vi "Sampling to Loop ms.vi"(4 "Sampling Config":T1) -> (7 "Loop Timeout ms":i32)   [LabVIEW 2020, in "VolatusDAQ.lvlib"]
uses:
  VolatusDAQ.lvlib
  VolatusDAQConfig/Sampling Config.ctl
  VolatusDAQConfig/VolatusDAQConfig.lvlib
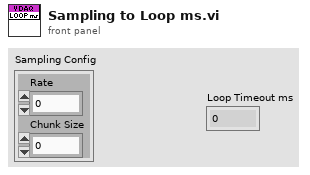
[diagram p1: front panel]
types:
  T1 = typedef "VolatusDAQConfig.lvlib/Sampling Config.ctl" = cluster{"Rate":dbl, "Chunk Size":i32}
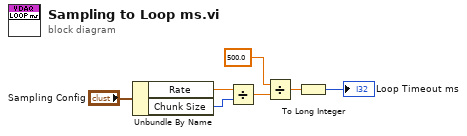
[diagram p0: block diagram]
diagram:
  n1 = Unbundle By Name("Sampling Config") -> ("Rate"=w7:dbl, "Chunk Size"=w6:i32)
  n2 = Divide(x=w7, y=w6) -> (x/y=w1:dbl)
  n3 = Divide(x=500.0 ("y"), y=w1) -> (x/y=w4:dbl)
  n4 = To Long Integer(number=w4) -> (32bit integer=→"Loop Timeout ms":i32)
